vi "Get CC Logics.vi"() -> ()   [LabVIEW 2015]
uses:
  Type/_RT Command.ctl
  <vilib>/Utility/config.llb/Read Key (U32).vi
  <vilib>/Utility/config.llb/Write Key (I32).vi
  <vilib>/Utility/config.llb/Write Key (U32).vi
  <vilib>/Utility/config.llb/NI_LVConfig.lvlib
panel:
  in  "LC2 Input Logics":enum32{"Shimadzu", "Others"}(radio)
  in  "LC1 Input Logics":enum32{"Shimadzu", "Others"}(radio)
  in  "LC-Hold Output Logics":enum32{"Shimadzu", "Others"}(radio)
  in  "Done":bool
  # "Please enter the logics for LC contact closure input and output"
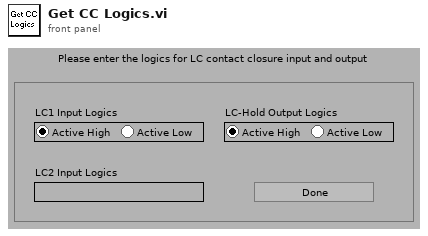
[diagram p1: front panel]
types:
  T1 = typedef "_RT Command.ctl" = enum16{"Start", "Stop", "Runtime Update", "Get Data", "Get Info", "Get Status", "Get Param", "Get Config", "Get Table", "Read ADC", "Set Oscillator", "Update Config", "Update Table", "Set All Pol", "Set Pol and DC", "Set Max Mass", "Toggle RP", "Toggle EL", "Set PIC", "Initialize Turbo", "Send Turbo Comm", "Close Turbo", "P1", "P2", "P3", "Send Serial", "Set LC Out", "Get LC In", "Read VAC", "Test Table", "Toggle Power", "Get Startup", "Set Startup", "Get ADC Table", "Set ADC Table", "Get Brief Status", "Get Detail Status", "Auxiliary Update", "Set CC Logics", "Set CC Input Logics", "Ignore Error"}
  T2 = typedef "NI_LVConfig.lvlib/Config Data RefNum.ctl" = refnum<k1>
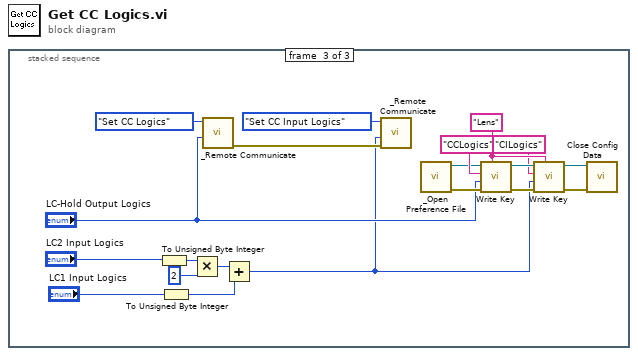
[diagram p0: block diagram]
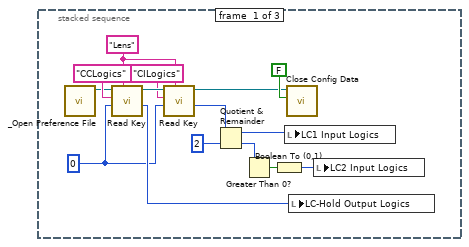
[diagram p2: hidden frame]
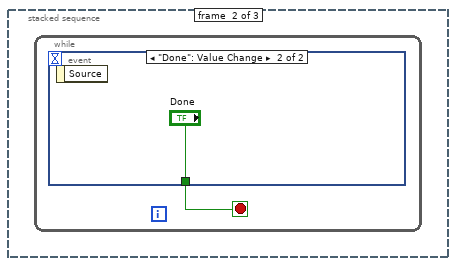
[diagram p3: hidden frame]
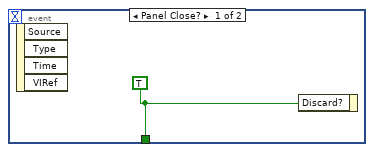
[diagram p4: hidden frame]
diagram:
  n1 = stacked-sequence {
    frame #0 {
      w8 = u8 0 ("y")
      w12 = "Lens" ("section")
      n2 = call "_Open Preference File.vi"() -> ("refnum"=w10:T2)  [unwired: 1 in, 6 out]
      n3 = call-poly <vilib>:"Read Key.vi"("section"=w12, "default value"=w8, "key"="CCLogics" ("section"), "refnum"=w10) -> ("value"=w9:u32, "refnum out"=w14:T2)  [unwired: 1 in, 5 out]
      n4 = call-poly <vilib>:"Read Key.vi"("section"=w12, "default value"=w8, "key"="CILogics" ("section"), "refnum"=w14) -> ("value"=w6:u32, "refnum out"=w7:T2)  [unwired: 1 in, 5 out]
      n5 = Quotient & Remainder(x=w6, y=u32 2) -> (x-y*floor(x/y)=w4:u32, floor(x/y)=w3:u32)
      n6 = Greater Than 0?(x=w3) -> (x > 0?=w2:bool)
      n7 = Boolean To (0,1)(Boolean=w2) -> (0, 1=w1:i16)
      n8 = local write "LC1 Input Logics"(w4) -> ()
      n9 = call <vilib>:"Close Config Data.vi"("write file if changed (T)"=FALSE ("write configuration file? (T)"), "refnum"=w7) -> ()  [unwired: 1 in, 9 out]
      n10 = local write "LC-Hold Output Logics"(w9) -> ()
      n11 = local write "LC2 Input Logics"(w1) -> ()
    }
    frame #1 {
      n12 = while {
        stop <- w16 stop-if-true
        n13 = event shown="[1] \"Done\": Value Change" {
          selector: _ -> [_ _]
          dyn-events: _ -> [_ _]
          timeout: _ -> [_ _]
          tunnel: [w17 "Done"] -> w16
          event Panel Close? {
            w17 = TRUE
            n14 = event-data() -> ()  [unwired: 5 out]
            n15 = event-data("Discard?"=w17) -> ()  [unwired: 1 in, 1 out]
          }
          event "Done": Value Change {
            n16 = event-data() -> ()  [unwired: 2 out]
          }
        }
      }
    }
    frame #2 {
      w26 = "Lens" ("section")
      n17 = To Unsigned Byte Integer(number="LC2 Input Logics") -> (unsigned 8bit integer=w38:u8)
      n18 = To Unsigned Byte Integer(number="LC1 Input Logics") -> (unsigned 8bit integer=w35:u8)
      n19 = Multiply(x=w38, y=u8 2) -> (x*y=w36:u8)
      n20 = call "_Remote Communicate.vi"("DC Param"="LC-Hold Output Logics", "Command"=_RT_Command."Set CC Logics") -> ("error out"=w30:errorcluster)  [unwired: 4 in, 3 out]
      n21 = Add(x=w36, y=w35) -> (x+y=w19:u8)
      n22 = call "_Remote Communicate.vi"("error in (no error)"=w30, "DC Param"=w19, "Command"=_RT_Command."Set CC Input Logics") -> ()  [unwired: 3 in, 4 out]
      n23 = call "_Open Preference File.vi"() -> ("error"=w21:errorcluster, "refnum"=w22:T2)  [unwired: 1 in, 5 out]
      n24 = call-poly <vilib>:"Write Key.vi"("section"=w26, "error in (no error)"=w21, "value"="LC-Hold Output Logics", "key"="CCLogics" ("section"), "refnum"=w22) -> ("error out"=w28:errorcluster, "refnum out"=w27:T2)  [unwired: 5 out]
      n25 = call-poly <vilib>:"Write Key.vi"("section"=w26, "error in (no error)"=w28, "value"=w19, "key"="CILogics" ("section"), "refnum"=w27) -> ("error out"=w23:errorcluster, "refnum out"=w24:T2)  [unwired: 5 out]
      n26 = call <vilib>:"Close Config Data.vi"("error in (no error)"=w23, "refnum"=w24) -> ()  [unwired: 1 in, 9 out]
    }
  }
